vi "02_表达式节点.vi"(10 "Temperature F1":dbl) -> (2 "Temperature C1":dbl)   [LabVIEW 2024]
doc: "本VI是为《我和LabVIEW》一书编写的示例。\n关于本书的介绍请参考网页：\nhttp://ruanqizhen.spaces.live.com/blog/cns!5852D4F797C53FB6!4310.entry"
panel:
  in  "stop":bool
  out "Temperature C2":dbl
  in  "Temperature F2":dbl
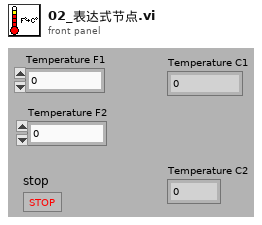
[diagram p1: front panel]
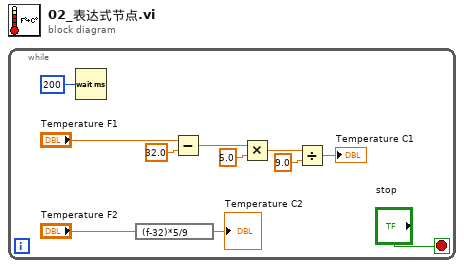
[diagram p0: block diagram]
diagram:
  n1 = while {
    stop <- "stop" stop-if-true
    n2 = Wait (ms)(milliseconds to wait=u32 200 ("millisecond timer value")) -> ()  [unwired: 1 out]
    n3 = expression code="(f-32)*5/9"("Temperature F2") -> (→"Temperature C2":dbl)
    n4 = Subtract(x="Temperature F1", y=32.0) -> (x-y=w11:dbl)
    n5 = Multiply(x=w11, y=5.0) -> (x*y=w10:dbl)
    n6 = Divide(x=w10, y=9.0) -> (x/y=→"Temperature C1":dbl)
  }
